vi "Configure Noise Source.vi"(8 "error in (no error)":errorcluster, 9 "Enable Noise Source (Disabled)":bool, 10 "Noise Source Type (1: Normal)":i32(ring)=1 items=["Smart Noise Source", "Normal"], 11 "VISA resource name":refnum<visa-resource-name>) -> (0 "error out":errorcluster, 3 "VISA resource name out":refnum<visa-resource-name>)   [LabVIEW 2014, in "Agilent ESA PSA Series.lvlib"]
doc: "Configures the source settings for the Noise Figure personality.\n\n<B>Note:</B> \n\nThis VI is only valid in Noise Figure personality. Use <B>Switch Personality</B> VI to switch to Noise Figure before calling this VI."
uses:
  Agilent ESA PSA Series.lvlib
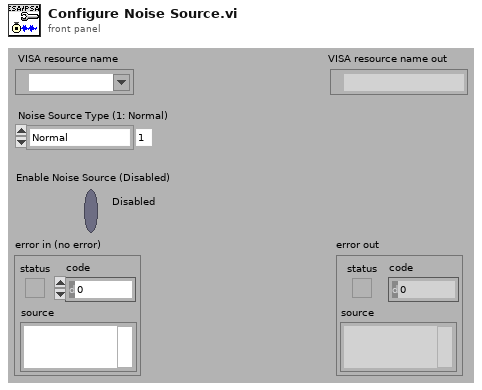
[diagram p1: front panel]
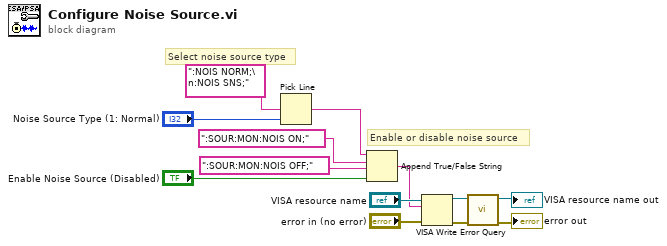
[diagram p0: block diagram]
diagram:
  # "Enable or disable noise source"
  # "Select noise source type"
  n1 = Pick Line(multi-line string=":NOIS NORM;\n:NOIS SNS;", line index="Noise Source Type (1: Normal)") -> (output string=w4:string)  [unwired: 1 in]
  n2 = Append True/False String(1:"Enable Noise Source (Disabled)", 2:":SOUR:MON:NOIS OFF;" ("false string"), 3:":SOUR:MON:NOIS ON;" ("true string"), 4:w4) -> (0:w1:string)
  n3 = VISA Write(VISA resource name="VISA resource name", write buffer=w1, error in (no error)="error in (no error)") -> (VISA resource name out=w11:refnum<visa-resource-name>, error out=w10:errorcluster)  [unwired: 1 out]
  n4 = call "Error Query.vi"("error in (no error)"=w10, "VISA resource name"=w11) -> ("error out"=→"error out":errorcluster, "VISA resource name out"=→"VISA resource name out":refnum<visa-resource-name>)  [unwired: 6 in, 2 out]
